vi "Lab2.vi"() -> ()   [LabVIEW 2019]
doc: "Simulator of heater model with PI controller, filter and datalogging"
uses:
  <vilib>/addons/WireFlow/_WireQueue/MQTT API/typedefs/MQTT_ConnectionDetails.ctl
  <vilib>/addons/WireFlow/_WireQueue/MQTT API/typedefs/MQTT_ComSetup.ctl
  <vilib>/addons/WireFlow/_WireQueue/MQTT API/typedefs/MQTT_ComType.ctl
  <vilib>/addons/WireFlow/_WireQueue/MQTT API/typedefs/MQTT_TLS-Conf.ctl
  <vilib>/Simulation/Scripting/Companion Diagram/SimConfigNode/SimParams.ctl
  <vilib>/Simulation/Scripting/Companion Diagram/SimConfigNode/_simSolvers.ctl
  <vilib>/Simulation/Implementation/Shared/SIMSCR Execution Mode.ctl
  <vilib>/Simulation/Param Hierarchy/Typedefs/SIMPH Param Control Actions.ctl
  <vilib>/Simulation/Implementation/Shared/NILVSim_ParamChanged.vi
  <vilib>/Simulation/Implementation/Shared/NILVSIM_BeginStep.vi
  <vilib>/Simulation/Implementation/Shared/NILVSim_Manager.vi
  <vilib>/Utility/error.llb/Clear Errors.vi
  <vilib>/Simulation/Implementation/Shared/NILVSim_FinalizeModel.vi
  <vilib>/Instr/_visa.llb/VISA Configure Serial Port (Instr).vi
  <vilib>/Simulation/Implementation/Shared/SIM Unbundle Sim Info.vi
  <vilib>/Simulation/Implementation/Shared/NILVSim_Initialize.vi
  <vilib>/Simulation/Utility/Implementation/NILVSim Get Time and IsAcceptedStep.vi
  <vilib>/Simulation/Implementation/Shared/SIMSH Read Queue.vi
  <vilib>/Simulation/Implementation/Shared/NILVSim_GetModelError.vi
  <vilib>/Simulation/Implementation/Shared/SIM Bundle Sim Info.vi
  <vilib>/Simulation/Implementation/XNodeFramework/SimXNode/SimX.xnode
  Air Heater Black Box Model.vi
  <vilib>/Simulation/Scripting/Companion Diagram/SimConfigNode/SimDog.xnode
  Sim with delay.vi
  <vilib>/Simulation/Implementation/Shared/NI_SIM_Implementation.lvlib
  <vilib>/addons/WireFlow/_WireQueue/MQTT API/MQTT_API.lvclass
panel:
  out "error out":errorcluster
  in  "error in":errorcluster
  in  "buffer size":u32=256
  in  "stop":bool
  out "Waveform Chart 2":dbl(graph)=1.1
  in  "Tab Control":T1(tab)
  in  "Temperature setpoint":dbl(knob)=28.0 scale=20.0..50.0
  in  "auto_man":bool=TRUE
  in  "man_output u [V]":dbl
  out "u":dbl=1.1
  in  "Ti":dbl=12.0 format="%.3f"
  in  "Kp":dbl=1.2 format="%.3f"
  out "y":dbl=25.067408902671477
  in  "Controller":string(combo)="LabVIEW"
  in  "Process Mode":string(combo)="Black Box"
  in  "Kh":dbl=3.5
  in  "theta_t":dbl=22.0
  in  "theta_d":dbl=2.0
  in  "T_env":dbl=21.0
  in  "baud rate":u32=4000000
  in  "data bits":u16=8 min=5 max=8 step=1
  in  "parity":u16(ring) items=["None", "Odd", "Even", "Mark", "Space"]
  in  "stop bits":u16=10
  in  "flow control":u16
  in  "timeout (ms)":u32=250
  in  "instr name":string="Arduino"
  out "status":bool
  out "read string":string="1.10\r\n"
  in  "MQTT String":string="field1=%.2f&field2=%.2f&field3=%.2f&field4=%.2f&field5=%.2f"
  in  "MQTT Topic":string="channels/1183879/publish/6NS6CK6FYU9IYVPA"
  out "Waveform Chart":T2(graph)={"Temperature setpoint"=25.0, "T_env"=25.067408902671477, "T_out"=0.0}
  # "Auto"
  # "Man"
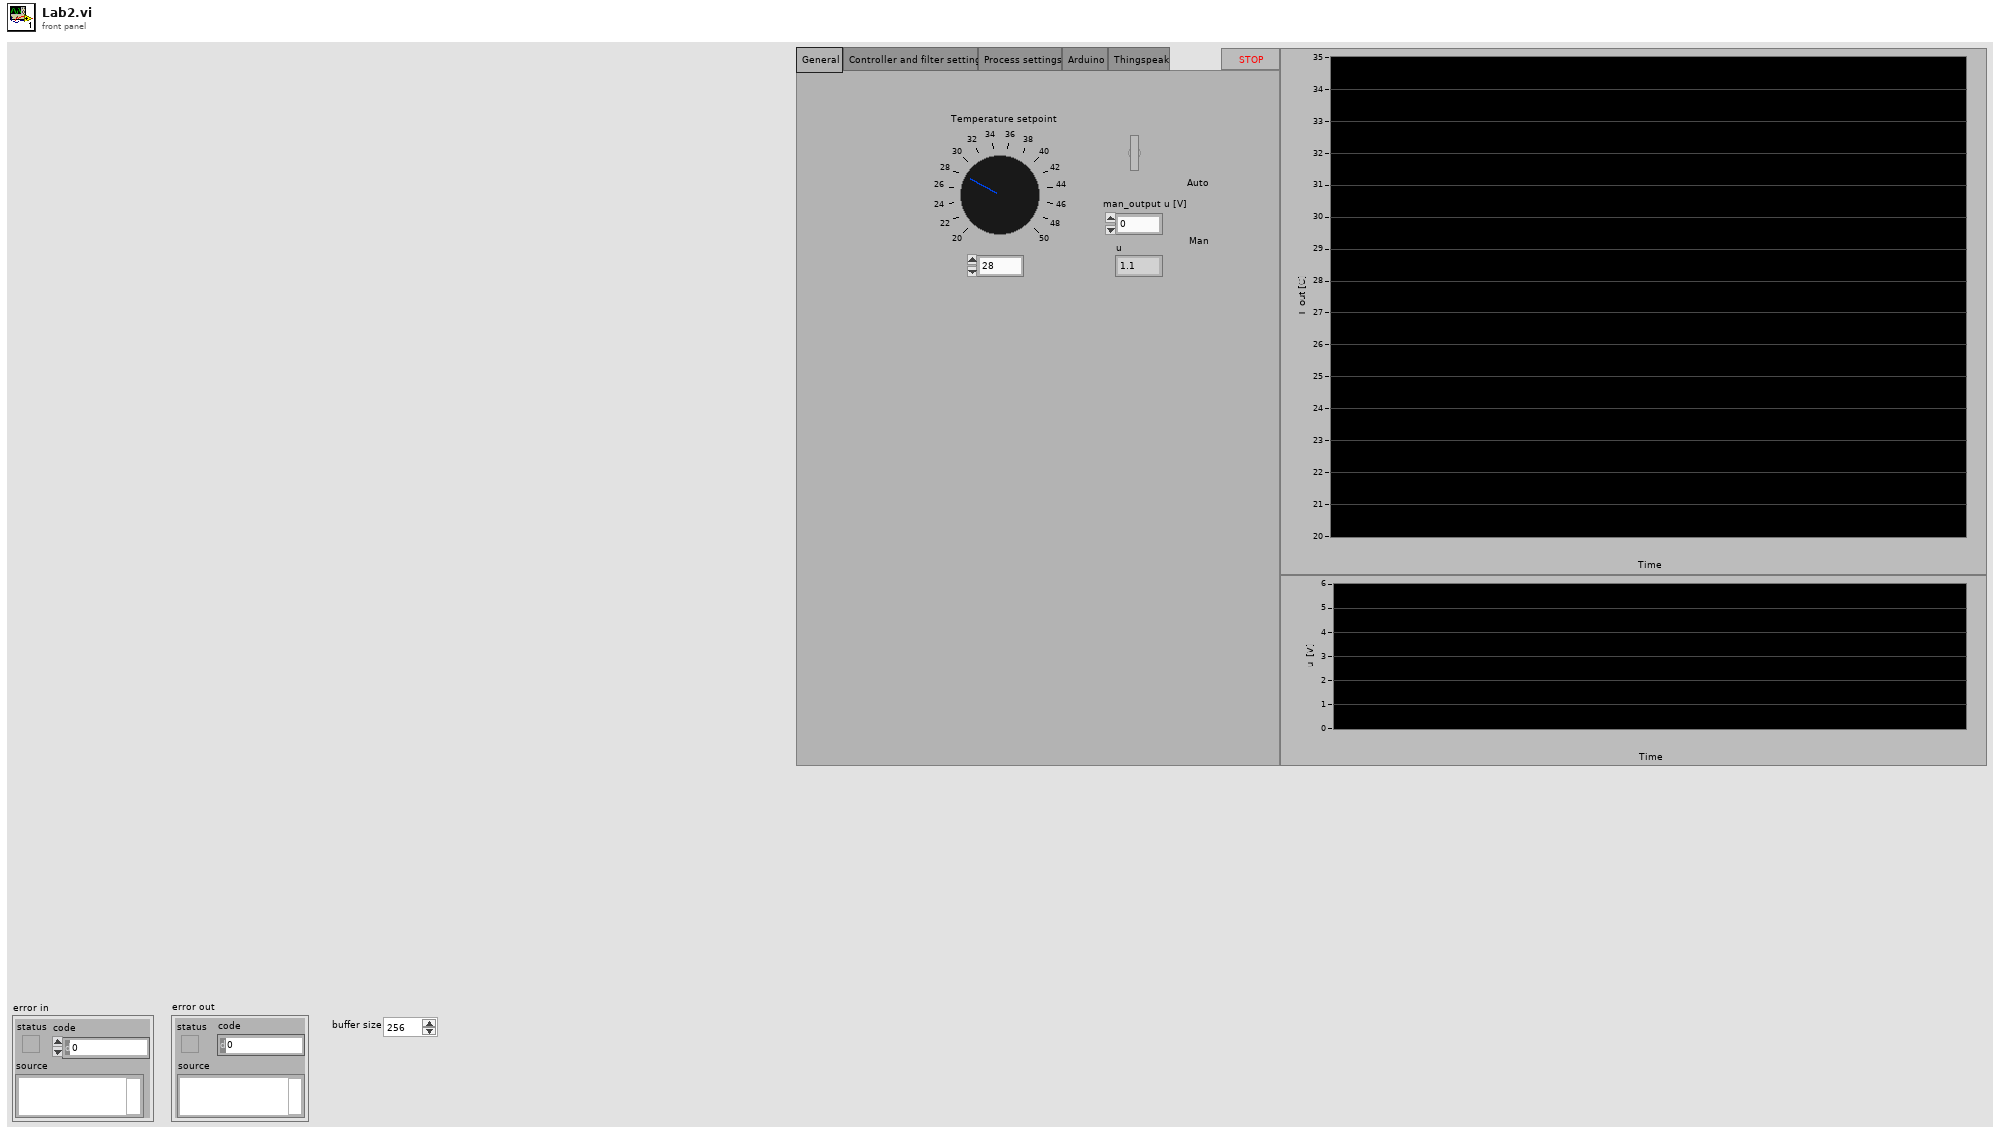
[diagram p1: front panel]
types:
  T1 = enum32{"General", "Controller and filter settings", "Process settings", "Arduino", "Thingspeak"}
  T2 = cluster{"Temperature setpoint":dbl, "T_env":dbl, "T_out":dbl}
  T3 = cluster{"Temperature setpoint":dbl, "T_env":dbl, "T_out":dbl}[]
  T4 = typedef "WF_WireQueue-MQTT.lvlib/MQTT_API.lvclass/MQTT_ComSetup.ctl" = cluster{"Communication type":T5, "TLS level (Full TLS)":T6, "TCP_NO-DELAY":bool}
  T5 = typedef "WF_WireQueue-MQTT.lvlib/MQTT_API.lvclass/MQTT_ComType.ctl" = enum16{"TCP/IP", "TCP/IP (TLS)"}
  T6 = typedef "WF_WireQueue-MQTT.lvlib/MQTT_API.lvclass/MQTT_TLS-Conf.ctl" = enum16{"Allow Self-signed crt", "Don't check server name", "Full TLS check"}
  T7 = typedef "WF_WireQueue-MQTT.lvlib/MQTT_API.lvclass/MQTT_ConnectionDetails.ctl" = cluster{"Server address":string, "Server port":u16, "User name":string, "Password":string, "Keep alive time (10 s)":u16, "Reconnect period (20 s)":u16, "Clean session reconnect?":bool}
  T8 = enum16{"Simulate to Completion", "Single Time-Step Simulation (Fixed Step Only)"}
  T9 = typedef "SIMSCR Execution Mode.ctl" = enum16{"Simulate to Completion", "Single Time-Step Simulation (Fixed Step Only)"}
  T10 = typedef "SIMPH Param Control Actions.ctl" = enum16{"get params", "set params"}
  T11 = cluster{"SIMSH Sim Time":dbl, "Select":cluster{"s? t:f":dbl}, "Linear Scaling with Points.vi":cluster{"y":dbl}, "Summation 3":cluster{"Result":dbl}, "Square Root":cluster{"sqrt(x)":dbl}, "Gaussian White Noise PtByPt.vi":cluster{"Gaussian white noise":dbl}, "Integrator":cluster{"output":dbl}, "Multiplication":cluster{"Result":dbl}, "Summation":cluster{"Result":dbl}, "Multiplication 2":cluster{"Result":dbl}, "Transport Delay":cluster{"output":dbl}, "Summation 2":cluster{"Result":dbl}}
  T12 = typedef "SimParams.ctl" = cluster{"Initial Time (s)":dbl, "Final Time (s)":dbl, "Step Size (s)":dbl, "ODE Solver":T13, "Minimum Step Size (s)":dbl, "Maximum Step Size (s)":dbl, "Relative Tolerance":dbl, "Absolute Tolerance":dbl, "Software Timing":bool, "Initial Step Size (s)":dbl, "Automatic Fixed Step Size?":bool, "Automatic Discrete Step Size?":bool, "Discrete Step Size (s)":dbl, "Calculate using Time Step":bool, "Solver Wired?":bool, "Prev.Frm.Expected End":u64, "Prev.Frm.Actual End":u64, "Prev.Frm.Finished Late?":bool, "Prev.Iter.Expected End":u64, "Prev.Iter.Actual End":u64, "Prev.Iter.Finished Late?":bool, "Expected Iteration Start":u64, "Actual Iteration Start":u64, "Expected Frame Start":u64, "Actual Frame Start":u64, "Source Name":string, "Name":string, "Period":i64, "Deadline":i64, "Offset":i64, "Start":i64, "Priority":i32, "Timeout":i32, "Processor":i32, "Mode":enum32{"No Change", "Process missed periods, maintain original phase", "Discard missed periods, maintain original phase", "Process missed periods, ignore original phase", "Discard missed periods, ignore original phase"}, "Wakeup reason":enum32{"Normal", "Aborted", "Asynchronous wakeup", "Timing source error", "Timed loop error", "Timeout"}, "Error":errorcluster, "Source Type":string, "Secondary Source Type":string, "Global End Time":u64, "Global Start Time":u64, "Full Solver Reset":bool, "Execution Mode":T9, "Nan/Inf Check":bool, "Custom Solver Library":string, "Solver Is Variable":bool, "custom solver name":string, "Signal Collection Decimation":u32}
  T13 = typedef "_simSolvers.ctl" = enum16{"Runge-Kutta 1 (Euler)", "Runge-Kutta 2", "Runge-Kutta 3", "Runge-Kutta 4", "Runge-Kutta 23 (variable)", "Runge-Kutta 45 (variable)", "BDF (variable)", "Adams-Moulton (variable)", "Rosenbrock (variable)", "Discrete States Only", "SDIRK 4 (variable)", "Radau 5 (variable)", "Radau 9 (variable)", "Radau 13 (variable)", "Radau [Variable Order] (variable)", "Gear's Method (variable)", "Linearizer", "State Query", "Trim Eval", "Custom Solver"}
  T14 = cluster{"SIMSH Sim Time":dbl, "upper limit":dbl, "Integrator":cluster{"output":dbl}, "Multiplication 2":cluster{"Result":dbl}, "Summation 2":cluster{"Result":dbl}, "Summation":cluster{"Result":dbl}, "Multiplication":cluster{"Result":dbl}, "Transport Delay":cluster{"output":dbl}}
  T15 = cluster{"Temperature setpoint":dbl, "Filter Output":dbl, "Tf [s]":dbl}
  T16 = cluster{"Temperature setpoint":dbl, "Filter Output":dbl, "T_out":dbl}
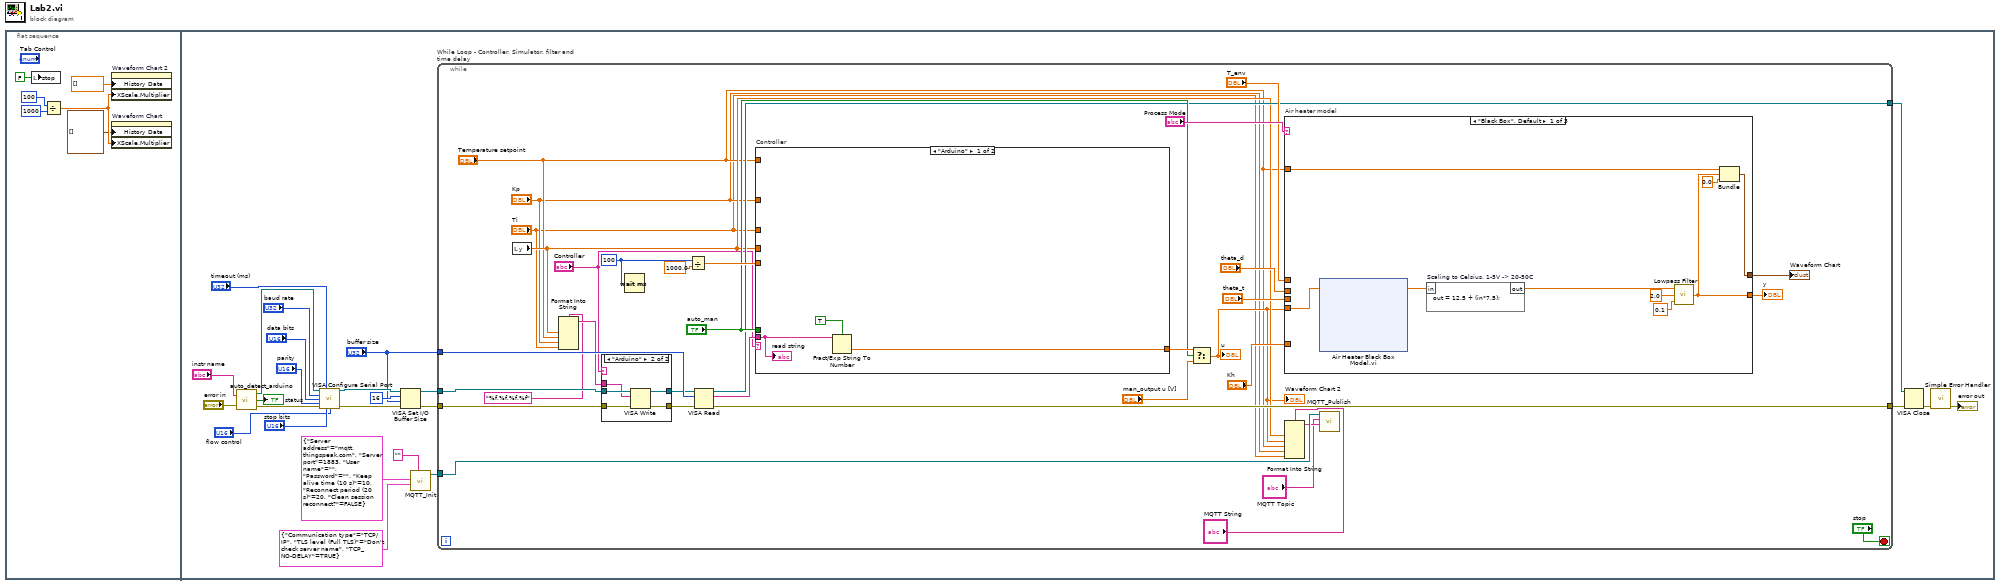
[diagram p0: block diagram]
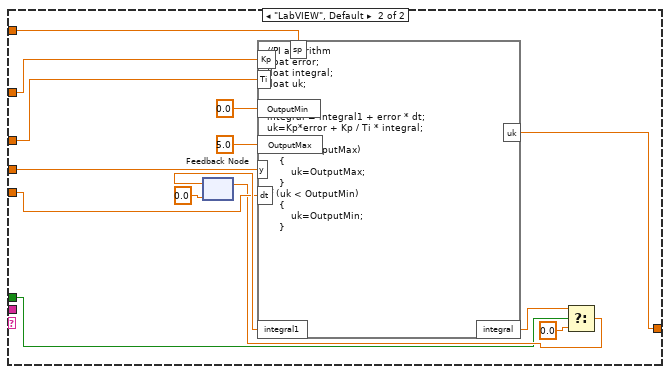
[diagram p2: hidden frame]
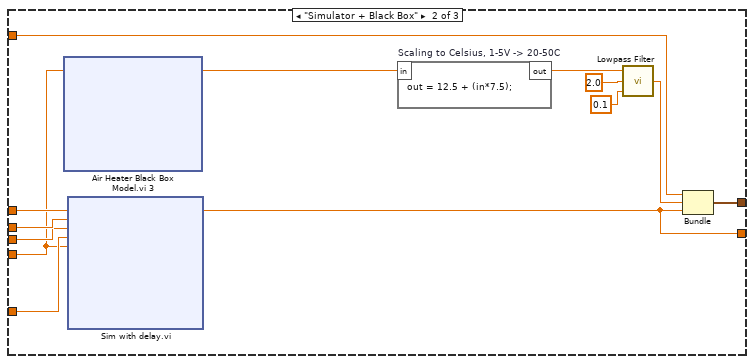
[diagram p4: hidden frame]
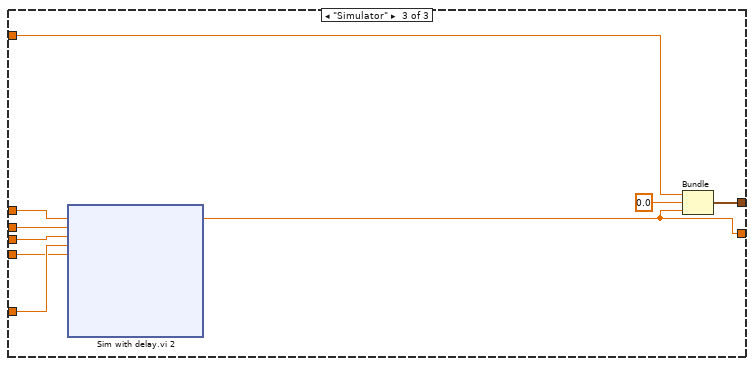
[diagram p5: hidden frame]
diagram:
  n1 = flat-sequence {
    frame #0 {
      n2 = local write "stop"(FALSE ("stop")) -> ()
      n3 = Divide(x=u32 100 ("milliseconds to wait"), y=u32 1000 ("x")) -> (x/y=w3:dbl)
      n4 = property on="Waveform Chart 2" class="WFChart (strict)"("History Data"=dbl[] [], "XScale.Multiplier"=w3) -> ()  [unwired: 2 in, 2 out]
      n5 = property on="Waveform Chart" class="WFChart (strict)"("History Data"=T3 [], "XScale.Multiplier"=w3) -> ()  [unwired: 2 in, 2 out]
    }
    frame #1 {
      n6 = call "auto_detect_arduino.vi"("instr name"="instr name", "error in"="error in") -> ("VISA resource name"=w25:refnum<visa-resource-name>, "status"=→"status":bool, "error out"=w26:errorcluster)
      n7 = call-poly "VISA Configure Serial Port"("VISA resource name"=w25, "timeout (10sec)"="timeout (ms)", "baud rate (9600)"="baud rate", "data bits (8)"="data bits", "parity (0:none)"="parity", "error in (no error)"=w26, "stop bits (10: 1 bit)"="stop bits", "flow control (0:none)"="flow control") -> ("VISA resource name out"=w28:refnum<visa-resource-name>, "error out"=w29:errorcluster)  [unwired: 6 in]
      n8 = VISA Set I/O Buffer Size(VISA resource name=w28, mask (16)=u16 16 ("I/O Receive\nBuffer mask"), size (4096)="buffer size", error in (no error)=w29) -> (VISA resource name out=w16:refnum<visa-resource-name>, error out=w17:errorcluster)
      n9 = call <vilib>:"MQTT_Init.vi"("Client ID"="", "Communication setup"=T4 {"Communication type"=enum."TCP/IP", "TLS level (Full TLS)"=enum."Don't check server name", "TCP_NO-DELAY"=TRUE}, "Connection details"=T7 {"Server address"="mqtt.thingspeak.com", "Server port"=1883, "User name"="", "Password"="", "Keep alive time (10 s)"=10, "Reconnect period (20 s)"=20, "Clean session reconnect?"=FALSE}) -> ("MQTT in"=w10:refnum<class "MQTT_API.lvclass">)  [unwired: 7 in, 1 out]
      n10 = while "While Loop - Controller, Simulator, filter and time delay" {
        tunnel: w17 -> [w52]
        tunnel: w16 -> [w53]
        tunnel: "buffer size" -> [w54]
        tunnel: [w51] -> w12
        tunnel: [w42] -> w11
        tunnel: w10 -> [w40]
        stop <- "stop" stop-if-true
        w57 = u32 100 ("milliseconds to wait")
        n11 = local read "y"() -> (w39:dbl)
        n12 = Format Into String(format string="%f,%f,%f,%f", w39, "Temperature setpoint", "Kp", "Ti") -> (resulting string=w49:string)  [unwired: 2 in, 1 out]
        n13 = case shown="\"Arduino\"" "Controller" {
          tunnel: w53 -> [w84 w89]
          tunnel: w52 -> [w83 w88]
          tunnel: [w84 w87] -> w50
          tunnel: [w83 w86] -> w55
          tunnel: w49 -> [_ w85]
          frame "LabView", Default {
          }
          frame "Arduino" {
            n14 = VISA Write(VISA resource name=w89, write buffer=w85, error in (no error)=w88) -> (VISA resource name out=w87:refnum<visa-resource-name>, error out=w86:errorcluster)  [unwired: 1 out]
          }
        }
        n15 = Wait (ms)(milliseconds to wait=w57) -> ()  [unwired: 1 out]
        n16 = Divide(x=w57, y=1000.0) -> (x/y=w47:dbl)
        n17 = VISA Read(VISA resource name=w50, byte count=w54, error in (no error)=w55) -> (VISA resource name out=w42:refnum<visa-resource-name>, read buffer=w43:string, error out=w51:errorcluster)  [unwired: 1 out]
        n18 = case "Controller" shown="\"Arduino\"" "Controller" {
          tunnel: "Kp" -> [_ w78]
          tunnel: "Ti" -> [_ w77]
          tunnel: w39 -> [_ w74]
          tunnel: w47 -> [_ w73]
          tunnel: "Temperature setpoint" -> [_ w72]
          tunnel: [w68 w70] -> w46
          tunnel: "auto_man" -> [_ w69]
          tunnel: w43 -> [w67 _]
          frame "Arduino" {
            n19 = Fract/Exp String To Number(use system decimal point (T)=TRUE, string=w67) -> (number=w68:dbl)  [unwired: 2 in, 1 out]
            "read string" <- w67
          }
          frame "LabVIEW", Default {
            n20 = feedback #1(0.0) -> (w81:dbl)
            n21 = formula code="//PI algorithm\nfloat error;\nfloat integral;\nfloat uk;\n\nerror=sp-y;\nintegral = integral1 + error * dt;\nuk=Kp*error + Kp / Ti * integral;\n\nif (uk > OutputMax)\n    {\n        uk=OutputMax;\n    }\nif (uk < OutputMin)\n    {\n        uk=OutputMin;\n    }"("Kp"=w78, "Ti"=w77, "OutputMin"=0.0 ("input variable"), "OutputMax"=5.0 ("input variable"), "y"=w74, "dt"=w73, "integral1"=w81, "sp"=w72) -> ("uk"=w70:dbl, "integral"=w82:dbl)
            n22 = Select(t=w82, s=w69, f=0.0) -> (s? t:f=w71:dbl)
            n23 = feedback-in #1(w71) -> ()
          }
        }
        n24 = Select(t=w46, s="auto_man", f="man_output u [V]") -> (s? t:f=w38:dbl)
        "Waveform Chart 2" <- w38
        "u" <- w38
        n25 = case "Air heater model" shown="\"Black Box\", Default" "Process Mode" {
          tunnel: [w93 w344 w868] -> w56
          tunnel: w38 -> [w91 w345 w869]
          tunnel: [w95 w352 w876] -> w64
          tunnel: "Kh" -> [_ w346 w870]
          tunnel: "T_env" -> [_ w349 w873]
          tunnel: "theta_d" -> [_ w348 w872]
          tunnel: "theta_t" -> [_ w347 w871]
          tunnel: "Temperature setpoint" -> [w92 w351 w874]
          frame "Black Box", Default {
            n26 = xnode "Air Heater Black Box Model.vi"("Control Signal [0-5V]"=w91) -> ("Tout [1-5V]"=w90:dbl)  [unwired: 2 in, 1 out]
            n27 = formula code="out = 12.5 + (in*7.5);" "Scaling to Celsius, 1-5V -> 20-50C"("in"=w90) -> ("out"=w98:dbl)
            n28 = call "Lowpass Filter.vi"("Ts [s]"=0.1, "Tf [s]"=2.0, "Filter Input"=w98) -> ("Filter Output"=w93:dbl)
            n29 = Bundle("Temperature setpoint"=w92, "Filter Output"=w93, "Tf [s]"=0.0) -> (w95:T15)  [unwired: 1 in]
          }
          frame "Simulator + Black Box" {
            n30 = xnode "Air Heater Black Box Model.vi 3"("Control Signal [0-5V]"=w345) -> ("Tout [1-5V]"=w350:dbl)  [unwired: 2 in, 1 out]
            n31 = xnode "Sim with delay.vi"("T_env"=w349, "theta_d"=w348, "theta_t"=w347, "Kh"=w346, "u"=w345) -> ("T_out"=w344:dbl)  [unwired: 2 in, 7 out]
            n32 = formula code="out = 12.5 + (in*7.5);" "Scaling to Celsius, 1-5V -> 20-50C"("in"=w350) -> ("out"=w356:dbl)
            n33 = call "Lowpass Filter.vi"("Ts [s]"=0.1, "Tf [s]"=2.0, "Filter Input"=w356) -> ("Filter Output"=w353:dbl)
            n34 = Bundle("Temperature setpoint"=w351, "Filter Output"=w353, "T_out"=w344) -> (w352:T16)  [unwired: 1 in]
          }
          frame "Simulator" {
            n35 = xnode "Sim with delay.vi 2"("T_env"=w873, "theta_d"=w872, "theta_t"=w871, "Kh"=w870, "u"=w869) -> ("T_out"=w868:dbl)  [unwired: 2 in, 7 out]
            n36 = Bundle("Temperature setpoint"=w874, "T_env"=0.0, "T_out"=w868) -> (w876:T2)  [unwired: 1 in]
          }
        }
        "Waveform Chart" <- w64
        "y" <- w56
        n37 = Format Into String(format string="MQTT String", w39, w38, "Temperature setpoint", "Kp", "Ti") -> (resulting string=w34:string)  [unwired: 2 in, 1 out]
        n38 = call <vilib>:"MQTT_Publish.vi"("Value"=w34, "Topic name"="MQTT Topic", "MQTT in"=w40) -> ()  [unwired: 7 in, 2 out]
      }
      n39 = VISA Close(VISA resource name=w11, error in (no error)=w12) -> (error out=w13:errorcluster)
      n40 = call <vilib>:"Simple Error Handler.vi"("error in (no error)"=w13) -> ("error out"=→"error out":errorcluster)  [unwired: 4 in, 4 out]
    }
  }
